vi "Create Evaluations.vi"(8 "error in (no error)":errorcluster, 11 "IEvaluation in":refnum<class "WCDMA_CHP.lvclass">) -> (0 "error out":errorcluster, 2 "Evaluations Out":T1[](array[typedef]) {"Low Limit" format="%#_13g"; "SI Scaling" items=["femto"=-15, "pico"=-12, "nano"=-9, "micro"=-6, "milli"=-3, "percent"=-2, ""=0, "kilo"=3, "mega"=6, "giga"=9, "tera"=12]}, 3 "IEvaluation out":refnum<class "WCDMA_CHP.lvclass">)   [LabVIEW 2016, in "SeqAuto Evaluations.lvlib" / "WCDMA_CHP.lvclass"]
uses:
  WCDMA_CHP.lvclass
  C:/projects/STS/Common/Sequence Automation/Plugins/SeqAuto IEvaluation.lvlibp/SeqAuto IEvaluation.lvclass
  Plugins/TestStand API Tools (TSAT).lvlibp/Evaluation Actions/Includes/Controls/TSAT Evaluation.ctl
  Plugins/TestStand API Tools (TSAT).lvlibp/Evaluation Actions/Includes/Controls/TSAT Eval SI Unit Scaling.ctl
  Plugins/TestStand API Tools (TSAT).lvlibp/Evaluation Actions/Includes/Controls/TSAT Evaluation Type.ctl
  WCDMA_CHP.lvclass/WCDMA_CHP.ctl
  Read SA Pin.vi
  Plugins/SeqAuto IEvaluation.lvlibp/Read Measurement Name.vi
  Plugins/TestStand API Tools (TSAT).lvlibp/Evaluation Actions/TSAT Evaluation Actions.lvlib
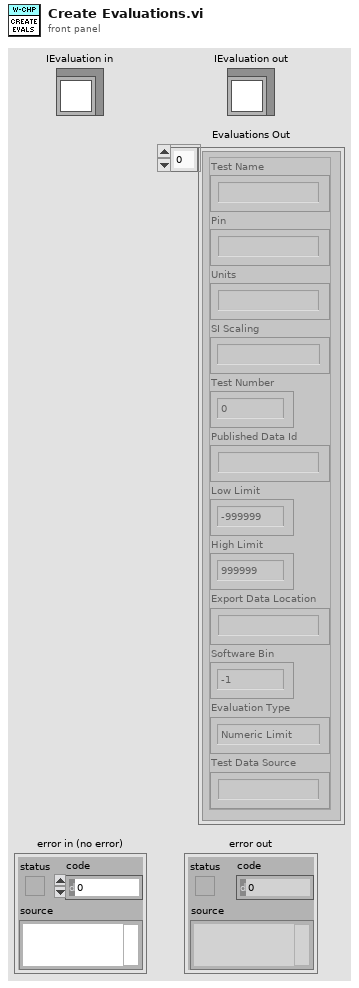
[diagram p1: front panel]
types:
  T1 = typedef "TestStand API Tools (TSAT).lvlibp/TSAT Evaluation Actions.lvlib/TSAT Evaluation.ctl" = cluster{"Test Name":string, "Pin":string, "Units":string, "SI Scaling":T2, "Test Number":i32, "Published Data Id":string, "Low Limit":dbl, "High Limit":dbl, "Export Data Location":string, "Software Bin":i64, "Evaluation Type":T3, "Test Data Source":string}
  T2 = typedef "TestStand API Tools (TSAT).lvlibp/TSAT Evaluation Actions.lvlib/TSAT Eval SI Unit Scaling.ctl" = i16
  T3 = typedef "TestStand API Tools (TSAT).lvlibp/TSAT Evaluation Actions.lvlib/TSAT Evaluation Type.ctl" = enum16{"Numeric Limit", "Pass/Fail", "None"}
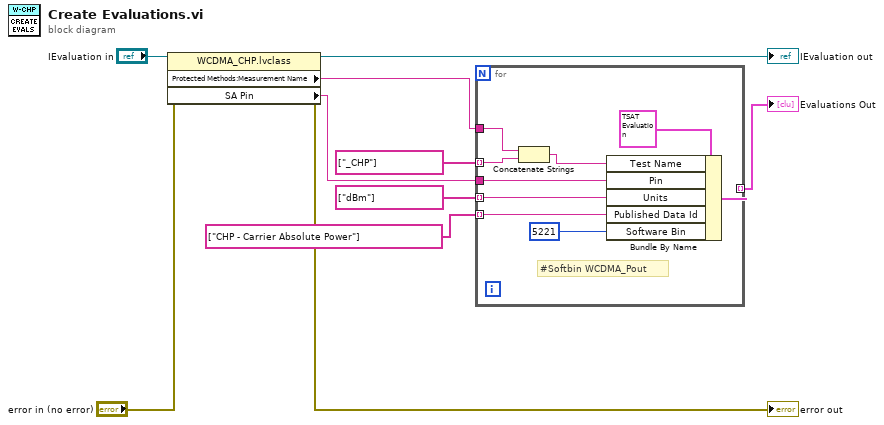
[diagram p0: block diagram]
diagram:
  n1 = property class="WCDMA_CHP.lvclass"(reference="IEvaluation in", error in="error in (no error)") -> (reference out=→"IEvaluation out":refnum<class "WCDMA_CHP.lvclass">, error out=→"error out":errorcluster, "Protected Methods:Measurement Name"=w6:string, "SA Pin"=w1:string)
  n2 = for {
    tunnel: [w18] -> w9 mode=indexing
    tunnel: w6 -> [w16]
    tunnel: string[] ["_CHP"] -> [w17] mode=indexing
    tunnel: string[] ["dBm"] -> [w14] mode=indexing
    tunnel: string[] ["CHP - Carrier Absolute Power"] -> [w13] mode=indexing
    tunnel: w1 -> [w12]
    # "#Softbin WCDMA_Pout"
    n3 = Concatenate Strings(w16, w17) -> (w15:string)
    n4 = Bundle By Name(cluster=T1 {"Test Name"="", "Pin"="", "Units"="", "SI Scaling"=0, "Test Number"=0, "Published Data Id"="", "Low Limit"=-999999.0, "High Limit"=999999.0, "Export Data Location"="", "Software Bin"=-1, "Evaluation Type"=enum."Numeric Limit", "Test Data Source"=""} ("Evaluation"), "Test Name"=w15, "Pin"=w12, "Units"=w14, "Published Data Id"=w13, "Software Bin"=i64 5221) -> (w18:T1)
  }
  "Evaluations Out" <- w9
